vi "wait for GFG variable change.vi"(8 "error in":errorcluster, 10 "Initialization Value":variant, 11 "Variable Name in":string="file.path") -> (0 "error out":errorcluster)   [LabVIEW 2012]
doc: "SciScan 1.2 160622"
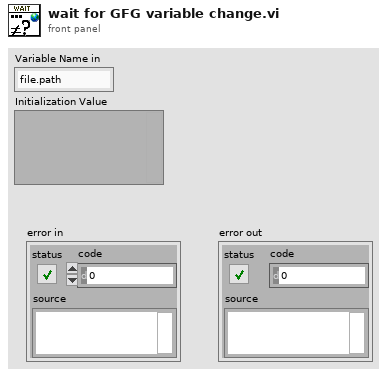
[diagram p1: front panel]
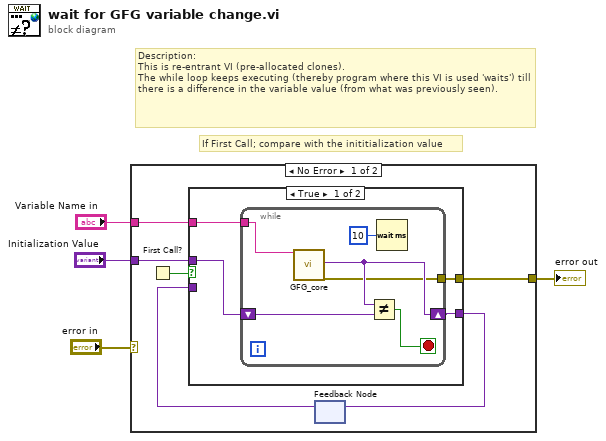
[diagram p0: block diagram]
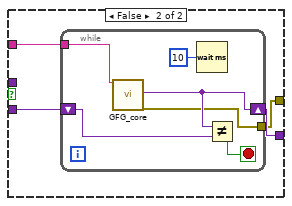
[diagram p2: hidden frame]
diagram:
  # "Description:\nThis is re-entrant VI (pre-allocated clones).\nThe while loop keeps executing (thereby program where this VI is used 'waits') till there is a difference in the variable value (from what was previously seen)."
  # "If First Call; compare with the inititialization value"
  n1 = case shown="No Error" "error in" {
    selector: "error in" -> [_ w31]
    tunnel: "Variable Name in" -> [w7 _]
    tunnel: "Initialization Value" -> [w6 _]
    tunnel: [w5 w31] -> w2
    frame No Error {
      n2 = First Call?() -> (First Call?: T/F=w8:bool)
      n3 = feedback #1() -> (w10:variant)  [unwired: 1 in]
      n4 = case shown="True" w8 {
        tunnel: [w14 w24] -> w9
        tunnel: w10 -> [_ w23]
        tunnel: w7 -> [w13 w22]
        tunnel: w6 -> [w12 _]
        tunnel: [w11 w21] -> w5
        frame True {
          n5 = while {
            shift-right: [w16] -> w14
            shift-left: w12 -> [w19]
            tunnel: w13 -> [w17]
            tunnel: [w15] -> w11
            stop <- w20 stop-if-true
            n6 = call "GFG_core.vi"("Variable Name in"=w17) -> ("Variant Out"=w16:variant, "error out"=w15:errorcluster)  [unwired: 12 in, 5 out]
            n7 = Not Equal?(x=w16, y=w19) -> (x != y?=w20:bool)
            n8 = Wait (ms)(milliseconds to wait=u32 10) -> ()  [unwired: 1 out]
          }
        }
        frame False {
          n9 = while {
            shift-right: [w26] -> w24
            shift-left: w23 -> [w29]
            tunnel: w22 -> [w27]
            tunnel: [w25] -> w21
            stop <- w30 stop-if-true
            n10 = call "GFG_core.vi"("Variable Name in"=w27) -> ("Variant Out"=w26:variant, "error out"=w25:errorcluster)  [unwired: 12 in, 5 out]
            n11 = Wait (ms)(milliseconds to wait=u32 10) -> ()  [unwired: 1 out]
            n12 = Not Equal?(x=w26, y=w29) -> (x != y?=w30:bool)
          }
        }
      }
      n13 = feedback-in #1(w9) -> ()
    }
    frame Error {
    }
  }
  "error out" <- w2
